vi "Write Sondenmodell.Parameter.vi"(8 "error in (no error)":errorcluster, 10 "Sondenmodell.Parameter":T1, 11 "Sondenmodell in":refnum<class "Sondenmodell.lvclass">) -> (0 "error out":errorcluster, 3 "Sondenmodell out":refnum<class "Sondenmodell.lvclass">)   [LabVIEW 2016, in "Sondenmodell.lvclass"]
uses:
  Sondenmodell.lvclass
  Sondenmodell.lvclass/Sondenmodell.ctl
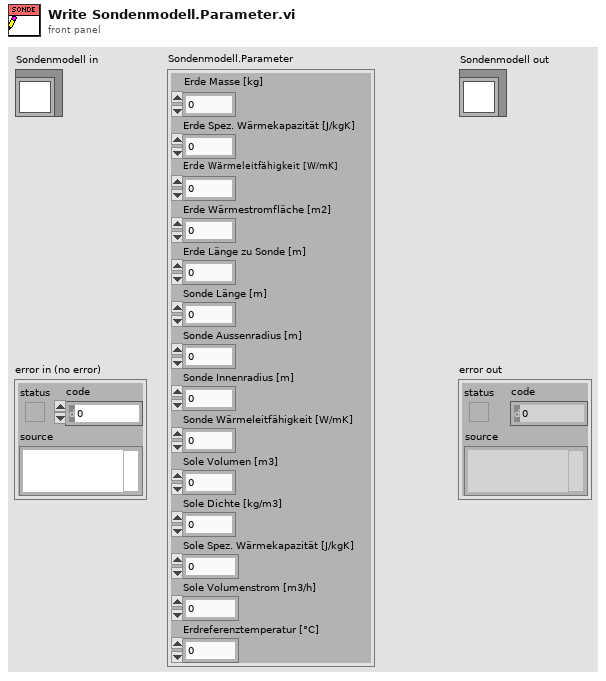
[diagram p1: front panel]
types:
  T1 = cluster{"Erde Masse [kg]":dbl, "Erde Spez. Wärmekapazität [J/kgK]":dbl, "Erde Wärmeleitfähigkeit [W/mK]":dbl, "Erde Wärmestromfläche [m2]":dbl, "Erde Länge zu Sonde [m]":dbl, "Sonde Länge [m]":dbl, "Sonde Aussenradius [m]":dbl, "Sonde Innenradius [m]":dbl, "Sonde Wärmeleitfähigkeit [W/mK]":dbl, "Sole Volumen [m3]":dbl, "Sole Dichte [kg/m3]":dbl, "Sole Spez. Wärmekapazität [J/kgK]":dbl, "Sole Volumenstrom [m3/h]":dbl, "Erdreferenztemperatur [°C]":dbl}
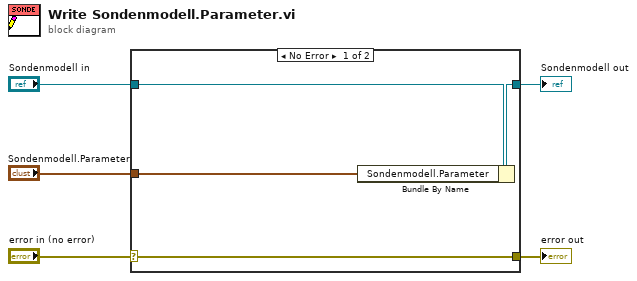
[diagram p0: block diagram]
diagram:
  n1 = case shown="No Error" "error in (no error)" {
    selector: "error in (no error)" -> [w9 w10]
    tunnel: [w9 w10] -> w4
    tunnel: [w7 w11] -> w2
    tunnel: "Sondenmodell in" -> [w8 w11]
    tunnel: "Sondenmodell.Parameter" -> [w6 _]
    frame No Error {
      n2 = Bundle By Name(cluster=w8, "Sondenmodell.Parameter"=w6) -> (w7:refnum<class "Sondenmodell.lvclass">)
    }
    frame Error {
    }
  }
  "error out" <- w4
  "Sondenmodell out" <- w2
